vi "SetMode.vi"(1 "Button":T1(ring), 2 "Mode":enum16{"Default", "Toggle"}(ring)) -> ()   [LabVIEW 2010, in "FTC.lvlib" / "Remote Interface.lvlib"]
uses:
  Remote Interface.lvlib
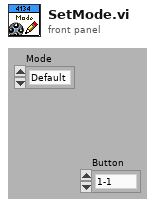
[diagram p1: front panel]
types:
  T1 = enum16{"1-1", "1-2", "1-3", "1-4", "1-5", "1-6", "1-7", "1-8", "1-9", "1-10", "1-11", "1-12", "2-1", "2-2", "2-3", "2-4", "2-5", "2-6", "2-7", "2-8", "2-9", "2-10", "2-11", "2-12", "NXT-L", "NXT-R", "NXT-E", "1-U", "1-UR", "1-R", "1-DR", "1-D", "1-DL", "1-L", "1-UL", "2-U", "2-UR", "2-R", "2-DR", "2-D", "2-DL", "2-L", "2-UL"}
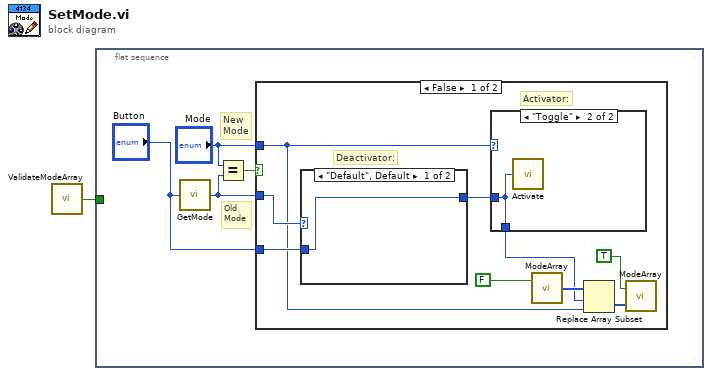
[diagram p0: block diagram]
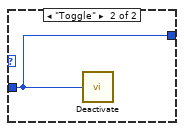
[diagram p2: hidden frame]
diagram:
  n1 = call "ValidateModeArray.vi"() -> ("Valid?"=w1:bool)
  n2 = flat-sequence {
    tunnel: w1 -> [_]
    frame #0 {
      # "New\nMode"
      # "Old\nMode"
      n3 = call "GetMode.vi"("Button"="Button") -> ("Mode"=w4:enum16{"Default", "Toggle"})
      n4 = Equal?(x="Mode", y=w4) -> (x = y?=w5:bool)
      n5 = case shown="False" w5 {
        tunnel: "Button" -> [w13 _]
        tunnel: w4 -> [w14 _]
        tunnel: "Mode" -> [w7 _]
        frame False {
          # "Activator:"
          # "Deactivator:"
          n6 = case shown="\"Default\", Default" w14 {
            tunnel: [w15 w16] -> w11
            tunnel: w13 -> [w15 w16]
            frame "Default", Default {
            }
            frame "Toggle" {
              n7 = call "Deactivate.vi"("Button"=w16) -> ()  [unwired: 1 in]
            }
          }
          n8 = case shown="\"Toggle\"" w7 {
            tunnel: w11 -> [w17 w18]
            tunnel: [w17 w18] -> w6
            frame "Default", Default {
            }
            frame "Toggle" {
              n9 = call "Activate.vi"("Button"=w18) -> ()  [unwired: 1 out]
            }
          }
          n10 = call "ModeArray.vi"("Write?"=FALSE) -> ("Array"=w12:u16[])  [unwired: 1 in]
          n11 = Replace Array Subset(array=w12, new element=w7, index=w6) -> (w8:u16[])
          n12 = call "ModeArray.vi"("Write Array"=w8, "Write?"=TRUE) -> ()  [unwired: 1 out]
        }
        frame True {
          # "No Change"
        }
      }
    }
  }
